vi "Register gRPC Methods.vi"(8 "error in (no error)":errorcluster, 11 "Template Server in":refnum<class "BLSPowerSupplyTemplateService.lvclass">) -> (0 "error out":errorcluster, 3 "Template Server out":refnum<class "BLSPowerSupplyTemplateService.lvclass">)   [LabVIEW 2023, in "BLSPowerSupplyTemplateService_server.lvlib" / "BLSPowerSupplyTemplateService.lvclass"]
uses:
  BLSPowerSupplyTemplateService.lvclass
  typeDefs/Server Internal UEs.ctl
  typeDefs/Server Internal Message.ctl
  typeDefs/Server gRPC UEs.ctl
  <vilib>/gRPC/LabVIEW gRPC Library/Server API/typeDefs/gRPCId Cluster.ctl
  <vilib>/gRPC/LabVIEW gRPC Library/Shared/grpcId.ctl
  BLSPowerSupplyTemplateService.lvclass/BLSPowerSupplyTemplateService.ctl
  <vilib>/gRPC/LabVIEW gRPC Library/grpc-lvsupport-release.lvlib
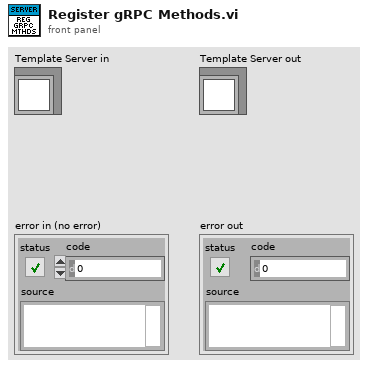
[diagram p1: front panel]
types:
  T1 = typedef "BLSPowerSupplyTemplateService_server.lvlib/BLSPowerSupplyTemplateService.lvclass/Server gRPC UEs.ctl" = cluster{"BLSPowerSupplyTemplateService SetNumber gRPC UE":refnum<user-event>}
  T2 = typedef "BLSPowerSupplyTemplateService_server.lvlib/BLSPowerSupplyTemplateService.lvclass/Server Internal UEs.ctl" = cluster{"BLSPowerSupplyTemplateService SetNumber Internal UE":refnum<user-event>}
  T3 = typedef "grpc-lvsupport-release.lvlib/grpcId.ctl" = u64
  T4 = typedef "BLSPowerSupplyTemplateService_server.lvlib/BLSPowerSupplyTemplateService.lvclass/Server Internal Message UE.ctl" = refnum<user-event>
  T5 = typedef "grpc-lvsupport-release.lvlib/gRPCId Cluster UE.ctl" = refnum<user-event>
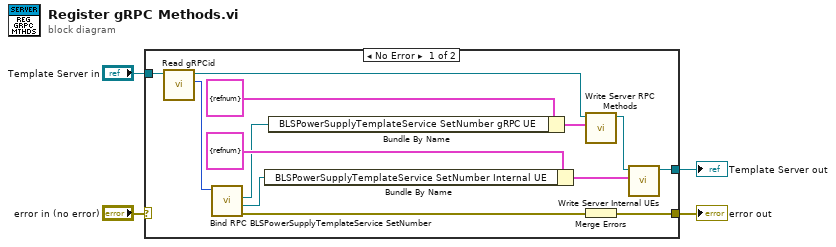
[diagram p0: block diagram]
diagram:
  n1 = case shown="No Error" "error in (no error)" {
    selector: "error in (no error)" -> [_ w18]
    tunnel: "Template Server in" -> [w9 w19]
    tunnel: [w17 w18] -> w3
    tunnel: [w16 w19] -> w2
    frame No Error {
      n2 = call-dynamic "Read gRPCid.vi"("iService in"=w9) -> ("gRPCid"=w8:T3, "iService out"=w10:refnum<class "BLSPowerSupplyTemplateService.lvclass">)  [unwired: 8 in, 1 out]
      n3 = call "Bind RPC BLSPowerSupplyTemplateService SetNumber.vi"("gRPCid server in"=w8) -> ("error out"=w7:errorcluster, "BLSPowerSupplyTemplateService SetNumber Internal UE"=w5:T4, "BLSPowerSupplyTemplateService SetNumber gRPC UE"=w6:T5)  [unwired: 7 in, 1 out]
      n4 = Bundle By Name ("Bundle Internal UEs")(cluster=T2 {"BLSPowerSupplyTemplateService SetNumber Internal UE"=refnum} ("Server Internal UEs"), "BLSPowerSupplyTemplateService SetNumber Internal UE"=w5) -> (w15:T2)
      n5 = Bundle By Name ("Bundle gRPC UEs")(cluster=T1 {"BLSPowerSupplyTemplateService SetNumber gRPC UE"=refnum} ("gRPC Server Method Events"), "BLSPowerSupplyTemplateService SetNumber gRPC UE"=w6) -> (w12:T1)
      n6 = call "Write Server RPC Methods.vi"("Server RPC Methods"=w12, "SignalGeneratorService in"=w10) -> ("SignalGeneratorService out"=w13:refnum<class "BLSPowerSupplyTemplateService.lvclass">)  [unwired: 8 in, 1 out]
      n7 = Merge Errors(w7) -> (w17:errorcluster)
      n8 = call "Write Server Internal UEs.vi"("Server Internal UEs"=w15, "SignalGeneratorService in"=w13) -> ("SignalGeneratorService out"=w16:refnum<class "BLSPowerSupplyTemplateService.lvclass">)  [unwired: 8 in, 1 out]
    }
    frame Error {
    }
  }
  "error out" <- w3
  "Template Server out" <- w2
